vi "HP53131 Measure Frequency2023.vi"(1 "GPIB Bus":i32=1 min=0 max=5, 3 "Number of Readings":i32=1 min=1, 4 "error in":errorcluster, 5 "GPIB Address":i16=10 max=31, 6 "Gate Time":dbl=1.0 min=0.0 max=1000.0 step=0.1 format="%.2f", 7 "Channel(1,2,3)":enum16{"Channel 1", "Channel 2", "Channel 3"}(ring)) -> (0 "error out":errorcluster, 2 "Frequency":dbl format="%.6f")   [LabVIEW 2024]
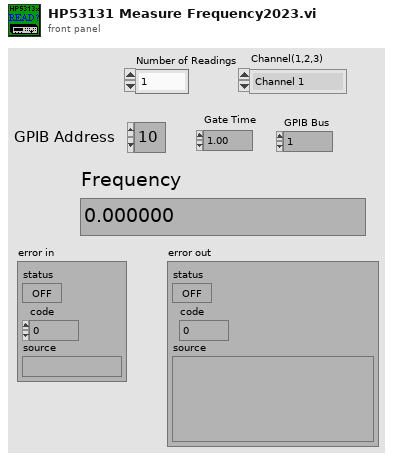
[diagram p1: front panel]
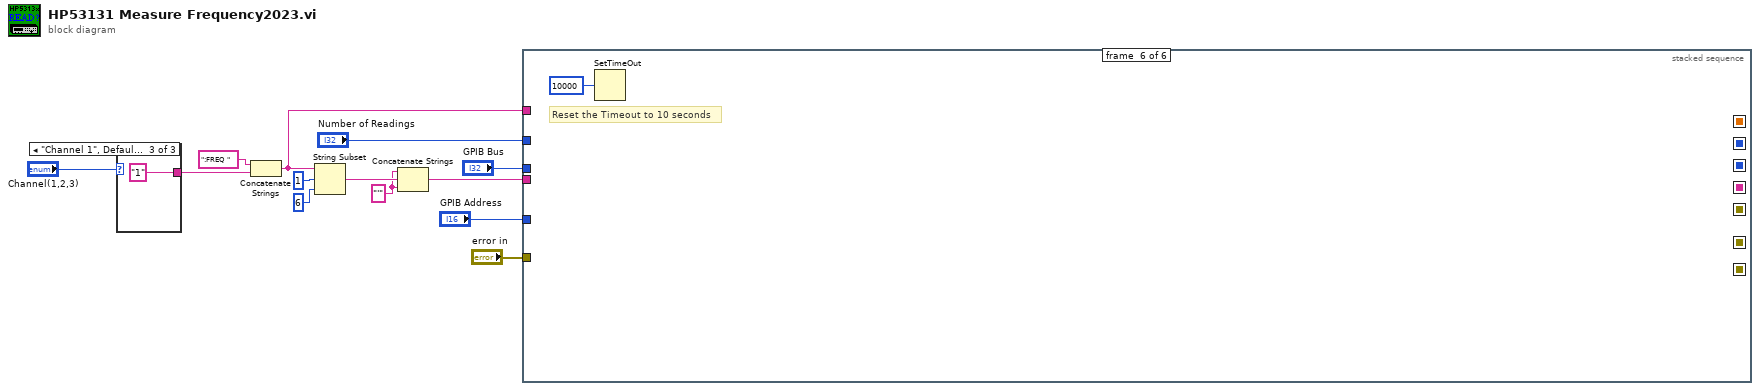
[diagram p0: block diagram]
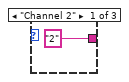
[diagram p2: hidden frame]
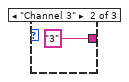
[diagram p3: hidden frame]
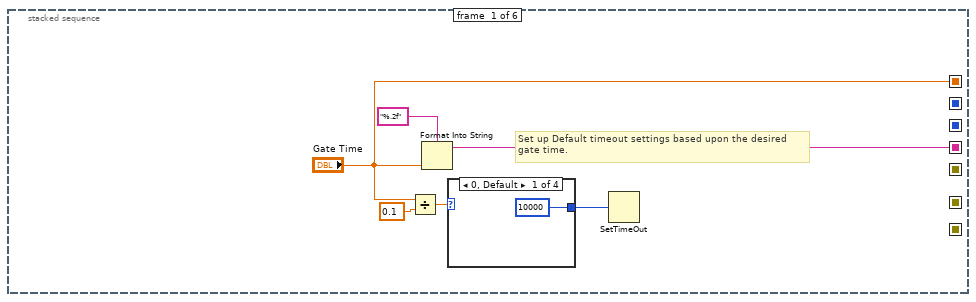
[diagram p4: hidden frame]
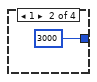
[diagram p5: hidden frame]
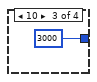
[diagram p6: hidden frame]
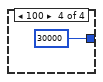
[diagram p7: hidden frame]
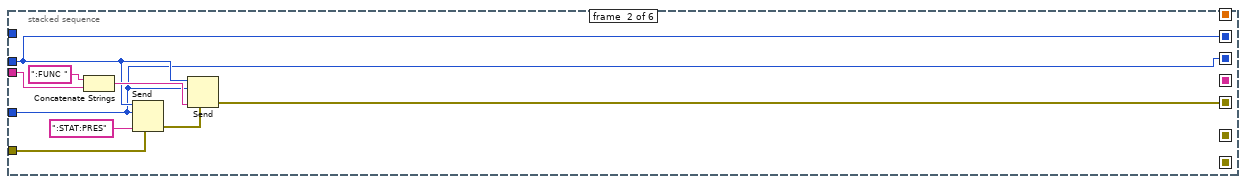
[diagram p8: hidden frame]
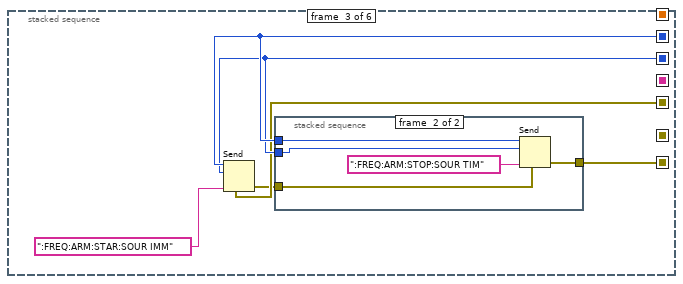
[diagram p9: hidden frame]
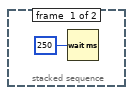
[diagram p10: hidden frame]
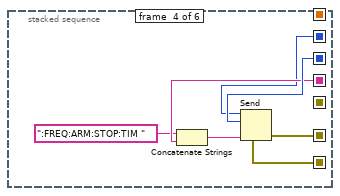
[diagram p11: hidden frame]
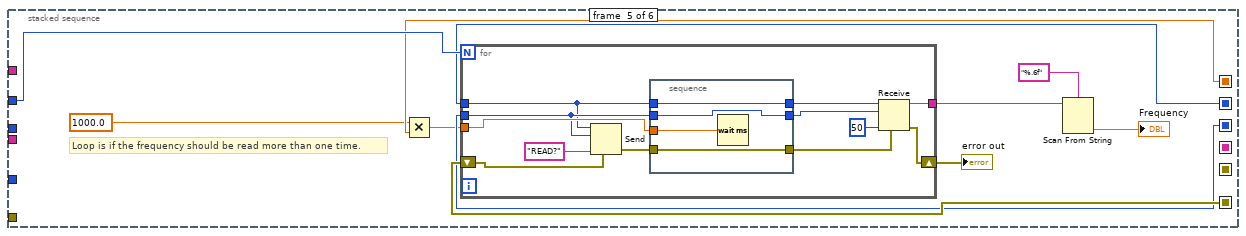
[diagram p12: hidden frame]
diagram:
  w4 = "'"
  n1 = case shown="\"Channel 1\", Default" "Channel(1,2,3)" {
    tunnel: ["2" "3" "1"] -> w10
    frame "Channel 2" {
    }
    frame "Channel 3" {
    }
    frame "Channel 1", Default {
    }
  }
  n2 = Concatenate Strings(":FREQ ", w10) -> (w8:string)
  n3 = String Subset(string=w8, offset (0)=1, length (rest)=6 ("length (rest)")) -> (substring=w5:string)
  n4 = Concatenate Strings(w4, w5, w4) -> (w3:string)
  n5 = stacked-sequence {
    seq-local: [_ w28 _ _ _ _] -> [_ _ w40 w54 w59 _]
    seq-local: [w21 _ _ _ _ _] -> [_ _ _ w52 _ _]
    seq-local: [_ w29 _ _ _ _] -> [_ _ w41 w51 w60 _]
    seq-local: [_ w34 _ _ _ _] -> [_ _ w39 _ _ _]
    seq-local: [_ _ w37 _ _ _] -> [_ _ _ w50 _ _]
    seq-local: [_ _ _ w49 _ _] -> [_ _ _ _ w62 _]
    seq-local: ["Gate Time" _ _ _ _ _] -> [_ _ _ _ w57 _]
    tunnel: "GPIB Address" -> [_ w28 _ _ _ _]
    tunnel: "GPIB Bus" -> [_ w29 _ _ _ _]
    tunnel: w8 -> [_ _ _ _ _ _]
    tunnel: w3 -> [_ w30 _ _ _ _]
    tunnel: "error in" -> [_ w27 _ _ _ _]
    tunnel: "Number of Readings" -> [_ _ _ _ w61 _]
    frame #0 {
      # "Set up Default timeout settings based upon the desired \ngate time."
      n6 = Divide(x="Gate Time", y=0.1) -> (x/y=w19:dbl)
      n7 = Format Into String(format string="%.2f" ("Format String"), "Gate Time") -> (resulting string=w21:string)  [unwired: 2 in, 1 out]
      n8 = case shown="0, Default" w19 {
        tunnel: [10000 3000 3000 30000] -> w20
        frame 0, Default {
        }
        frame 1 {
        }
        frame 10 {
        }
        frame 100 {
        }
      }
      n9 = SetTimeOut(1:w20) -> ()  [unwired: 1 out]
    }
    frame #1 {
      n10 = Concatenate Strings(":FUNC " ("data string"), w30) -> (w31:string)
      n11 = Send(0:w29, 2:w28, 4:w27, 5:":STAT:PRES" ("data string")) -> (8:w33:errorcluster)  [unwired: 1 in, 2 out]
      n12 = Send(0:w29, 2:w28, 4:w33, 5:w31) -> (8:w34:errorcluster)  [unwired: 1 in, 2 out]
    }
    frame #2 {
      n13 = Send(0:w41, 2:w40, 4:w39, 5:":FREQ:ARM:STAR:SOUR IMM" ("data string")) -> (8:w38:errorcluster)  [unwired: 1 in, 2 out]
      n14 = stacked-sequence {
        tunnel: w41 -> [_ w47]
        tunnel: w40 -> [_ w46]
        tunnel: w38 -> [_ w45]
        tunnel: [_ w44] -> w37
        frame #0 {
          n15 = Wait (ms)(milliseconds to wait=u32 250) -> ()  [unwired: 1 out]
        }
        frame #1 {
          n16 = Send(0:w47, 2:w46, 4:w45, 5:":FREQ:ARM:STOP:SOUR TIM" ("data string")) -> (8:w44:errorcluster)  [unwired: 1 in, 2 out]
        }
      }
    }
    frame #3 {
      n17 = Concatenate Strings(":FREQ:ARM:STOP:TIM " ("data string"), w52) -> (w53:string)
      n18 = Send(0:w51, 2:w54, 4:w50, 5:w53) -> (8:w49:errorcluster)  [unwired: 1 in, 2 out]
    }
    frame #4 {
      # "Loop is if the frequency should be read more than one time."
      n19 = Multiply(x=1000.0, y=w57) -> (x*y=w55:dbl)
      n20 = for {
        N: w61 -> [_]
        tunnel: w59 -> [w68]
        tunnel: w60 -> [w67]
        tunnel: [w76] -> w63
        shift-right: [w73] -> w58
        shift-left: w62 -> [w75]
        tunnel: w55 -> [w72]
        n21 = Send(0:w67, 2:w68, 4:w75, 5:"READ?" ("data string")) -> (8:w71:errorcluster)  [unwired: 1 in, 2 out]
        n22 = stacked-sequence {
          tunnel: w72 -> [w81]
          tunnel: w71 -> [w78]
          tunnel: [w79] -> w70
          tunnel: [w80] -> w69
          tunnel: w68 -> [w80]
          tunnel: w67 -> [w79]
          tunnel: [w78] -> w66
          frame #0 {
            n23 = Wait (ms)(milliseconds to wait=w81) -> ()  [unwired: 1 out]
          }
        }
        n24 = Receive(4:w66, 6:50 ("count"), 8:w69, 9:w70) -> (0:w73:errorcluster, 3:w76:string)  [unwired: 1 in, 2 out]
      }
      "error out" <- w58
      n25 = Scan From String(format string="%.6f" ("Format String"), input string=w63) -> (output 1=→"Frequency":dbl)  [unwired: 3 in, 3 out]
    }
    frame #5 {
      # "Reset the Timeout to 10 seconds"
      n26 = SetTimeOut(1:10000 ("new timeout (10000)")) -> ()  [unwired: 1 out]
    }
  }
